vi "Serial Port Flush.vi"(8 "error in (no error)":errorcluster, 11 "VISA resource name":refnum<visa-resource-name>="COM1") -> (0 "error out":errorcluster, 1 "FLUSHED CHARS":string, 3 "duplicate VISA resource name":refnum<visa-resource-name>)   [LabVIEW 2020]
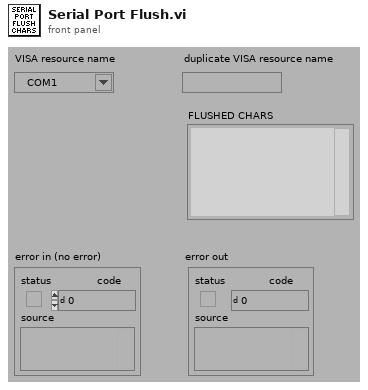
[diagram p1: front panel]
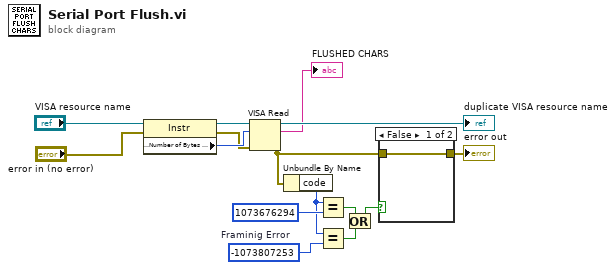
[diagram p0: block diagram]
diagram:
  w5 = -1073807253  # Framinig Error
  n1 = property class="Instr"(reference="VISA resource name", error in="error in (no error)") -> (reference out=w11:refnum<visa-resource-name>, error out=w13:errorcluster, "Serial Settings:Number of Bytes at Serial Port"=w14:u32)
  n2 = VISA Read(VISA resource name=w11, byte count=w14, error in (no error)=w13) -> (VISA resource name out=→"duplicate VISA resource name":refnum<visa-resource-name>, read buffer=→"FLUSHED CHARS":string, error out=w8:errorcluster)  [unwired: 1 out]
  n3 = Unbundle By Name(w8) -> ("code"=w4:i32)
  n4 = Equal?(x=w4, y=1073676294) -> (x = y?=w3:bool)
  n5 = Equal?(x=w4, y=w5) -> (x = y?=w2:bool)
  n6 = Or(x=w3, y=w2) -> (x .or. y?=w1:bool)
  n7 = case shown="False" w1 {
    tunnel: [w16 _] -> w9
    tunnel: w8 -> [w16 _]
    frame False {
    }
    frame True {
    }
  }
  "error out" <- w9
